vi "Test Configuration Files.vi"() -> ()   [LabVIEW 2018]
panel:
  out "AI":path
  out "Serial":path
  out "DI":path
  out "DO":path
  out "Command Data":string[](array[string])
  in  "Directory":path
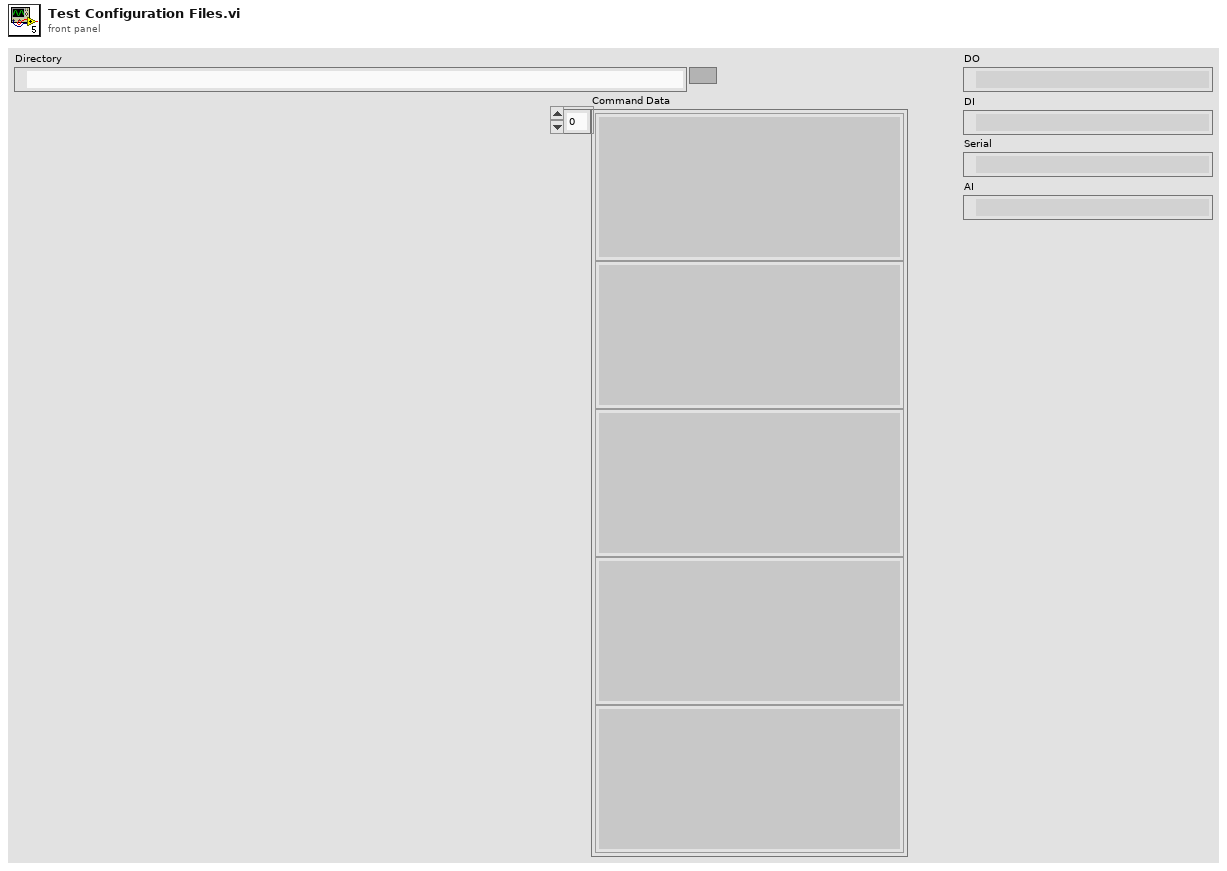
[diagram p1: front panel]
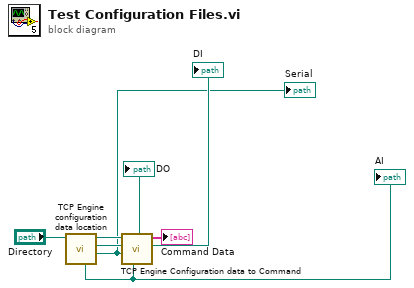
[diagram p0: block diagram]
diagram:
  n1 = call "TCP Engine configuration data location.vi"("Directory"="Directory") -> ("Serial"=w4:path, "DI"=w5:path, "DO"=w6:path, "AI"=w3:path)  [unwired: 7 in]
  "DO" <- w6
  "DI" <- w5
  "Serial" <- w4
  "AI" <- w3
  n2 = call "TCP Engine Configuration data to Command.vi"("AI"=w3, "Serial"=w4, "DI"=w5, "DO"=w6) -> ("Command Data"=→"Command Data":string[])  [unwired: 7 in]
